vi "My_DHT11_Labview1.vi"() -> ()   [LabVIEW 2024]
uses:
  <vilib>/Instr/_visa.llb/VISA Configure Serial Port (Instr).vi
panel:
  in  "Tab Control 2":enum32{"Hum Chart", "Hum Gauge"}(tab)
  out "Waveform Chart 2":dbl(graph)
  out "Gauge 2":dbl(knob) scale=0.0..100.0 scale format="%%%#_g"
  in  "Tab Control":enum32{"Temp Chart", "Temp Gauge"}(tab)
  out "Waveform Chart":dbl(graph)
  out "Gauge":dbl(knob) scale=0.0..50.0
  out "Fan LED 2":bool
  out "Fan LED":bool
  in  "Fan":bool
  out "Humidity":dbl(slide) scale=0.0..100.0 scale format="%%%d"
  out "Temperature":dbl(slide) scale=0.0..100.0
  in  "?":bool
  in  "VISA Arduino Uno":refnum<visa-resource-name>
  in  "Fan 2":bool
  # "Environmental Control System for Greenhouses\n\nMonitoring System"
  # "House No. 1"
  # "C"
  # "%"
  # "Eng. Yahia Gaddal\ngaddal18@gmail.com"
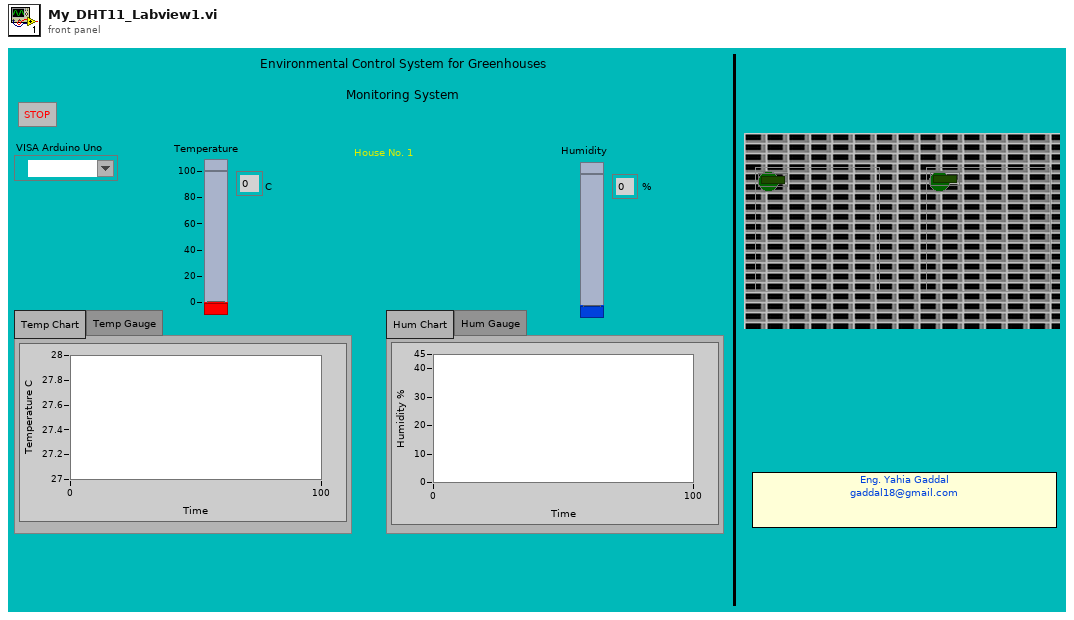
[diagram p1: front panel]
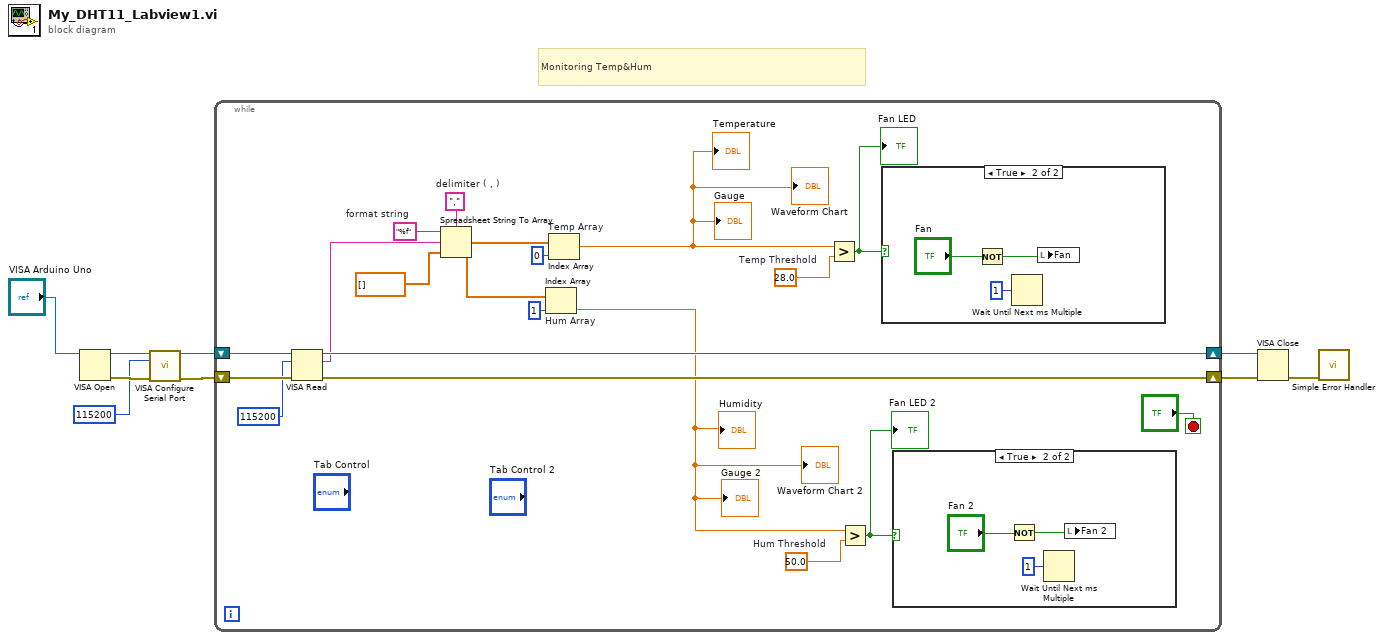
[diagram p0: block diagram]
diagram:
  # "Monitoring Temp&Hum"
  n1 = VISA Open(VISA resource name="VISA Arduino Uno") -> (VISA resource name=w9:refnum<visa-resource-name>, error out=w8:errorcluster)  [unwired: 4 in]
  n2 = call-poly "VISA Configure Serial Port"("VISA resource name"=w9, "baud rate (9600)"=u32 115200, "error in (no error)"=w8) -> ("VISA resource name out"=w7:refnum<visa-resource-name>, "error out"=w6:errorcluster)  [unwired: 11 in]
  n3 = while {
    shift-right: [w25] -> w5
    shift-left: w7 -> [w28]
    shift-right: [w24] -> w4
    shift-left: w6 -> [w27]
    stop <- "?" stop-if-true
    w13 = 50.0  # Hum Threshold
    w17 = ","  # delimiter ( , )
    w20 = "%f"  # format string
    w22 = 28.0  # Temp Threshold
    n4 = VISA Read(VISA resource name=w28, byte count=u32 115200, error in (no error)=w27) -> (VISA resource name out=w25:refnum<visa-resource-name>, read buffer=w19:string, error out=w24:errorcluster)  [unwired: 1 out]
    n5 = Spreadsheet String To Array(delimiter (Tab)=w17, format string=w20, spreadsheet string=w19, array type (2D Dbl)=dbl[] []) -> (array=w15:dbl[])
    n6 = Index Array "Hum Array"(array=w15, index=1) -> (element=w10:dbl)
    "Humidity" <- w10
    "Waveform Chart 2" <- w10
    "Gauge 2" <- w10
    n7 = Index Array "Temp Array"(array=w15, index=0) -> (element=w11:dbl)
    "Temperature" <- w11
    "Gauge" <- w11
    "Waveform Chart" <- w11
    n8 = Greater?(x=w11, y=w22) -> (0:w21:bool)
    "Fan LED" <- w21
    n9 = Greater?(x=w10, y=w13) -> (0:w12:bool)
    "Fan LED 2" <- w12
    n10 = case shown="True" w21 {
      frame False {
      }
      frame True {
        n11 = Not(x="Fan") -> (.not. x?=w33:bool)
        n12 = Wait Until Next ms Multiple(millisecond multiple=u32 1) -> ()  [unwired: 1 out]
        n13 = local write "Fan"(w33) -> ()
      }
    }
    n14 = case shown="True" w12 {
      frame False {
      }
      frame True {
        n15 = Not(x="Fan 2") -> (.not. x?=w29:bool)
        n16 = Wait Until Next ms Multiple(millisecond multiple=u32 1) -> ()  [unwired: 1 out]
        n17 = local write "Fan 2"(w29) -> ()
      }
    }
  }
  n18 = VISA Close(VISA resource name=w5, error in (no error)=w4) -> (error out=w1:errorcluster)
  n19 = call <vilib>:"Simple Error Handler.vi"("error in (no error)"=w1) -> ()  [unwired: 4 in, 5 out]
